vi "Parameters To Technique Parameters.vi"(8 "error in (no error)":errorcluster, 10 "Parameters":T1, 11 "ParameterIN":variant) -> (0 "error out":errorcluster, 3 "Params Values":T2[](array[typedef]))   [LabVIEW 2022 SP3, in "EClib functions.lvlib"]
uses:
  EClib functions.lvlib
  TechniqueParameters.ctl
  Parameters.ctl
  CAParameters.ctl
  CASGParameters.ctl
  CPParameters.ctl
  GEISParameters.ctl
  ISCANParameters.ctl
  OCVParameters.ctl
  PEISParameters.ctl
  SCCXParameters.ctl
  SGEISParameters.ctl
  SPEISParameters.ctl
  VSCANParameters.ctl
  MPParameters.ctl
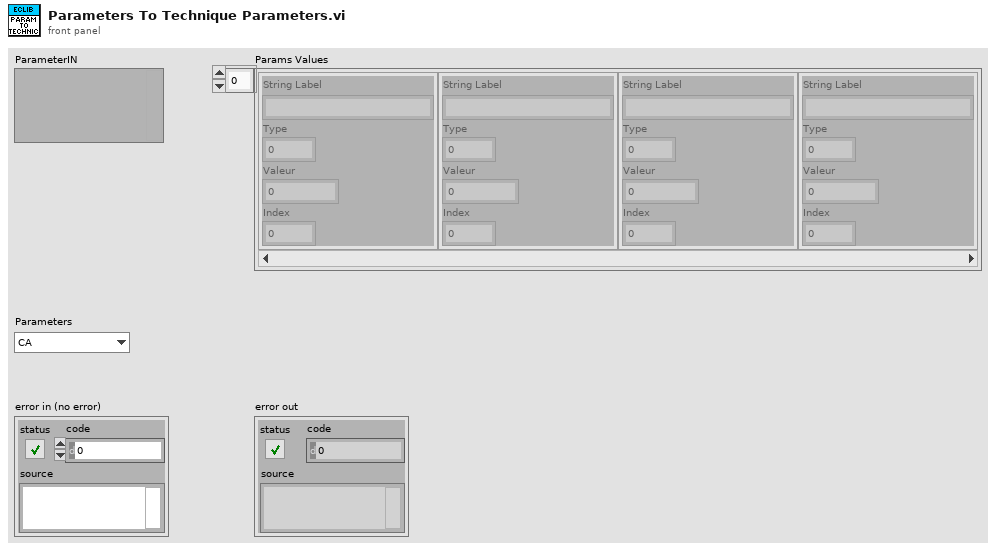
[diagram p1: front panel]
types:
  T1 = typedef "EClib functions.lvlib/Parameters.ctl" = enum16{"CA", "CASG", "CP", "GEIS", "ISCAN", "OCV", "PEIS", "SCCX", "SGEIS", "SPEIS", "VSCAN", "MP"}
  T2 = typedef "EClib functions.lvlib/TechniqueParameters.ctl" = cluster{"String Label":string, "Type":i32, "Valeur":i32, "Index":i32}
  T3 = typedef "EClib functions.lvlib/CAParameters.ctl" = cluster{"tb":sgl, "Steps":cluster{"vs_initial":bool, "Voltage_step":sgl, "Duration_step":sgl}[], "Step_number":i32, "N_Cycles":i32, "Record_every_dI":sgl, "Record_every_dT":sgl, "I_Range":u16, "E_Range":u16, "Bandwidth":u16, "em":u16, "ce":u16}
  T4 = typedef "EClib functions.lvlib/CASGParameters.ctl" = cluster{"Ii":sgl, "Ii_vs_initial":bool, "Steps":cluster{"I1_vs_initial":bool, "I1":sgl, "Period_number":u32, "Fs":sgl, "Record_every_dE":sgl, "Record_every_dT":sgl, "I2_vs_initial":bool, "I2":sgl}[], "Step_number":i32, "N_Cycles":i32, "I_Range":u16, "Bandwidth":u16, "em":u16, "ce":u16, "tb":sgl}
  T5 = typedef "EClib functions.lvlib/CPParameters.ctl" = cluster{"Steps":cluster{"vs_initial":bool, "Current_step":sgl, "Duration_step":sgl}[], "Step_number":i32, "N_Cycles":i32, "Record_every_dE":sgl, "Record_every_dT":sgl, "I_Range":u16, "E_Range":u16, "Bandwidth":u16, "em":u16, "ce":u16, "tb":sgl}
  T6 = typedef "EClib functions.lvlib/GEISParameters.ctl" = cluster{"Step_number":i32, "Initial_Current_step":sgl, "vs_initial ":bool, "Final_Current_step":sgl, "vs_final":bool, "Duration_step":sgl, "Record_every_dE":sgl, "Record_every_dT":sgl, "Initial_frequency":sgl, "sweep":bool, "Final_frequency":sgl, "Frequency_number":i32, "Amplitude_Current":sgl, "Wait_for_steady":sgl, "Average_N_times":i32, "Correction":bool, "I_Range":u16, "Bandwidth":u16, "em":u16, "ce":u16}
  T7 = typedef "EClib functions.lvlib/ISCANParameters.ctl" = cluster{"vs_initial ":bool, "Current_step":sgl, "Scans":cluster{" vs_initial":bool, "Current_step":sgl, "Scan_Rate":sgl}[], "Scan_number":i32, "N_Cycles":i32, "Record_every_dI":sgl, "Begin_measuring_E":sgl, "End_measuring_E":sgl, "I_Range":u16, "E_Range":u16, "Bandwidth":u16, "em":u16, "ce":u16, "tb":sgl}
  T8 = typedef "EClib functions.lvlib/OCVParameters.ctl" = cluster{"Rest_time_T":sgl, "Record_every_dE":sgl, "Record_every_dT":sgl, "E_Range":u16, "em":u16, "ce":u16, "tb":sgl}
  T9 = typedef "EClib functions.lvlib/PEISParameters.ctl" = cluster{"Step_number":i32, "Initial_Voltage_step":sgl, "vs_initial":bool, "Final_Voltage_step":sgl, "vs_final":bool, "Duration_step":sgl, "Record_every_dI":sgl, "Record_every_dT":sgl, "Initial_frequency":sgl, "sweep":bool, "Final_frequency":sgl, "Frequency_number":i32, "Amplitude_Voltage":sgl, "Wait_for_steady":sgl, "Average_N_times":i32, "Correction":bool, "I_Range":u16, "Bandwidth":u16, "em":u16, "ce":u16}
  T10 = typedef "EClib functions.lvlib/SCCXParameters.ctl" = cluster{"I_Range":u16, "E_Range":u16, "Bandwidth":u16, "par_E0":sgl, "par_A":sgl, "par_B":sgl, "par_QRP_select":u16, "par_E_duration":sgl, "par_E_dt_rec":sgl, "par_I0_duration":sgl, "par_I0_dt_rec":sgl, "par_NC":i32, "par_RC":i32, "par_Q_limit_val":sgl, "par_Q_limit_cfg":u16, "par_QRP_time":sgl, "ce":i32, "em":i32}
  T11 = cluster{"SCCX Parameters":T10, "Channel information":cluster{"Channel":i32, "BoardVersion":i32, "BoardSerialCode":i32, "FirmwareCode":i32, "FirmwareVersion":i32, "XilinxVersion":i32, "AmpCode":i32, "NbAmp":i32, "LcBoard":i32, "Zboard":i32, "MuxBoard":i32, "GPRAboard":i32, "MemSize":i32, "MemFilled":i32, "state":i32, "MaxIRange":i32, "MinIRange":i32, "MaxBandwidth":i32, "NbOfTechniques":i32}}
  T12 = typedef "EClib functions.lvlib/SGEISParameters.ctl" = cluster{"Step_number":i32, "Initial_Current_step":sgl, "vs_initial ":bool, "Final_Current_step":sgl, "vs_final":bool, "Duration_step":sgl, "Record_every_dE":sgl, "Record_every_dT":sgl, "Initial_frequency":sgl, "sweep":bool, "Final_frequency":sgl, "Frequency_number":i32, "Amplitude_Current":sgl, "Wait_for_steady":sgl, "Average_N_times":i32, "Correction":bool, "I_Range":u16, "Bandwidth":u16, "em":u16, "ce":u16}
  T13 = typedef "EClib functions.lvlib/SPEISParameters.ctl" = cluster{"Step_number":i32, "Initial_Voltage_step":sgl, "vs_initial":bool, "Final_Voltage_step":sgl, "vs_final":bool, "Duration_step":sgl, "Record_every_dI":sgl, "Record_every_dT":sgl, "Initial_frequency":sgl, "sweep":bool, "Final_frequency":sgl, "Frequency_number":i32, "Amplitude_Voltage":sgl, "Wait_for_steady":sgl, "Average_N_times":i32, "Correction":bool, "I_Range":u16, "Bandwidth":u16, "em":u16, "ce":u16}
  T14 = typedef "EClib functions.lvlib/VSCANParameters.ctl" = cluster{"tb":sgl, "vs_initial ":bool, "Voltage_step":sgl, "Scans":cluster{" vs_initial ":bool, "Voltage_step":sgl, "Scan_Rate":sgl}[], "Scan_number":i32, "N_Cycles":i32, "Record_every_dE":sgl, "Begin_measuring_I":sgl, "End_measuring_I":sgl, "I_Range":u16, "E_Range":u16, "Bandwidth":u16, "em":u16, "ce":u16}
  T15 = typedef "EClib functions.lvlib/MPParameters.ctl" = cluster{"tb":sgl, "Scans":cluster{"Value_step":sgl, "Duration_step":sgl, " vs_initial ":bool, "Record_every_dT":sgl, "Record_every_dM":sgl, "Mode_step":i32}[], "I_Range":u16, "Bandwidth":u16, "N_Cycles":i32, "Record_every_rc":i32, "ce":u16, "em":u16, "Step_number":i32}
  T16 = cluster{"I1_vs_initial":bool, "I1":sgl, "Period_number":u32, "Fs":sgl, "Record_every_dE":sgl, "Record_every_dT":sgl, "I2_vs_initial":bool, "I2":sgl}[]
  T17 = cluster{"I1_vs_initial":bool, "I1":sgl, "Period_number":u32, "Fs":sgl, "Record_every_dE":sgl, "Record_every_dT":sgl, "I2_vs_initial":bool, "I2":sgl}
  T18 = cluster{"Channel":i32, "BoardVersion":i32, "BoardSerialCode":i32, "FirmwareCode":i32, "FirmwareVersion":i32, "XilinxVersion":i32, "AmpCode":i32, "NbAmp":i32, "LcBoard":i32, "Zboard":i32, "MuxBoard":i32, "GPRAboard":i32, "MemSize":i32, "MemFilled":i32, "state":i32, "MaxIRange":i32, "MinIRange":i32, "MaxBandwidth":i32, "NbOfTechniques":i32}
  T19 = cluster{"Label":string, "type":i32, "valeur":u32, "index":i32}[]
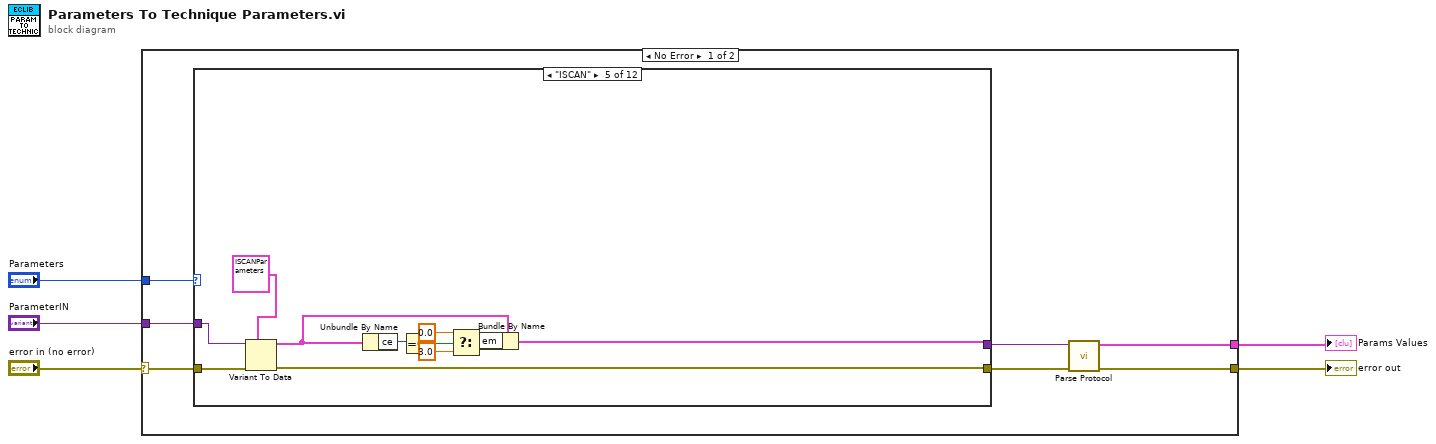
[diagram p0: block diagram]
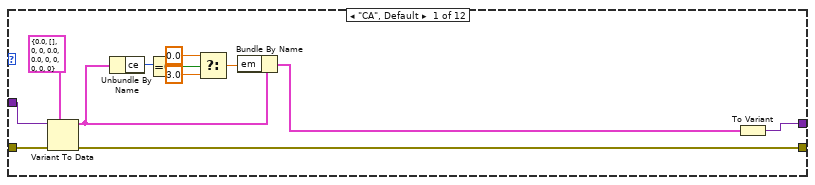
[diagram p2: hidden frame]
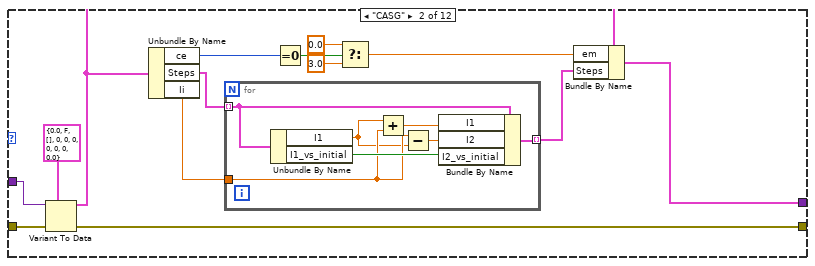
[diagram p3: hidden frame]
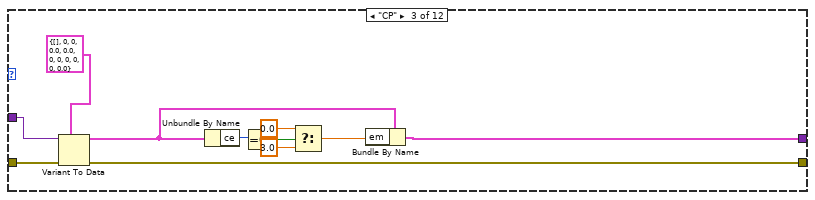
[diagram p4: hidden frame]
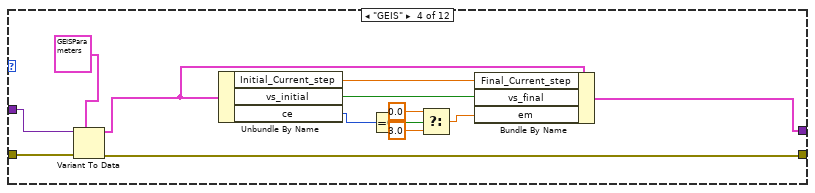
[diagram p5: hidden frame]
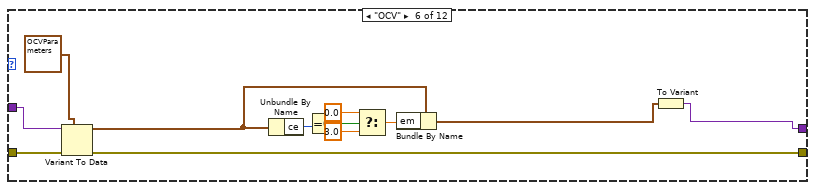
[diagram p6: hidden frame]
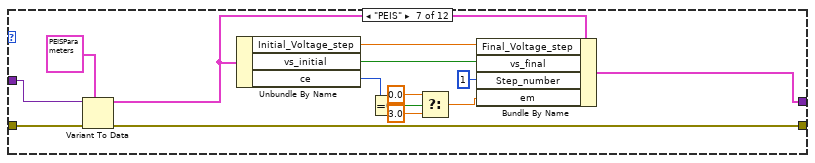
[diagram p7: hidden frame]
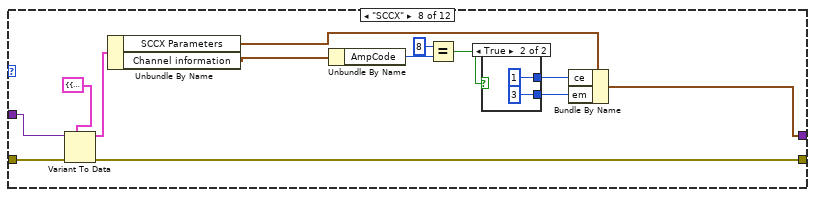
[diagram p8: hidden frame]
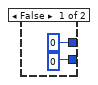
[diagram p9: hidden frame]
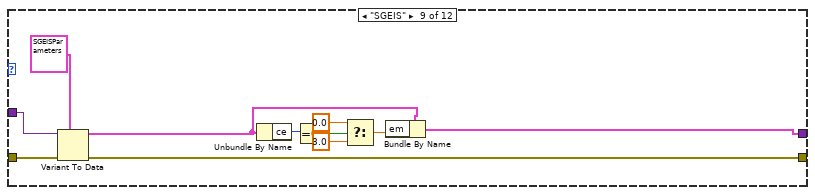
[diagram p10: hidden frame]
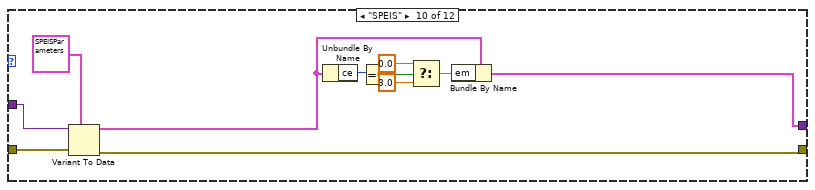
[diagram p11: hidden frame]
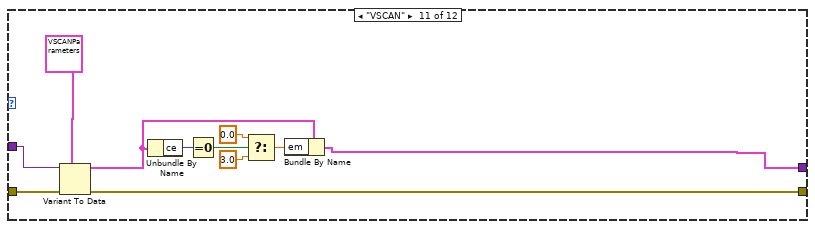
[diagram p12: hidden frame]
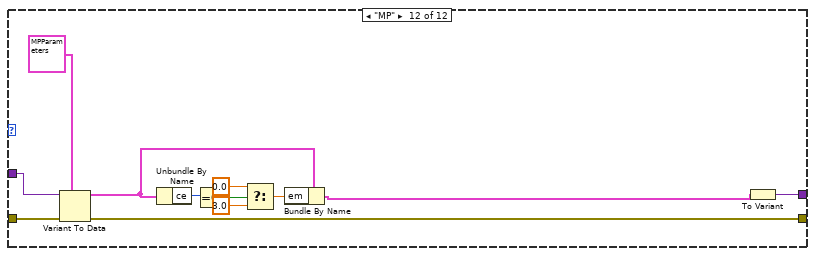
[diagram p13: hidden frame]
diagram:
  n1 = case shown="No Error" "error in (no error)" {
    selector: "error in (no error)" -> [w12 w169]
    tunnel: [w8 _] -> w5
    tunnel: [w6 w169] -> w3
    tunnel: "ParameterIN" -> [w10 _]
    tunnel: "Parameters" -> [w11 _]
    frame No Error {
      n2 = case shown="\"ISCAN\"" w11 {
        tunnel: [w14 w26 w47 w58 w70 w81 w94 w108 w124 w135 w146 w157] -> w9
        tunnel: w12 -> [w19 w38 w51 w69 w80 w92 w105 w119 w134 w145 w156 w168]
        tunnel: w10 -> [w17 w37 w50 w68 w79 w91 w106 w118 w133 w144 w155 w167]
        tunnel: [w13 w25 w46 w66 w77 w89 w93 w107 w132 w143 w147 w166] -> w7
        frame "CA", Default {
          n3 = Variant To Data(error in=w19, type=T3 {"tb"=0.0, "Steps"=[], "Step_number"=0, "N_Cycles"=0, "Record_every_dI"=0.0, "Record_every_dT"=0.0, "I_Range"=0, "E_Range"=0, "Bandwidth"=0, "em"=0, "ce"=0} ("CA Parameters"), Variant=w17) -> (data=w16:T3, error out=w13:errorcluster)
          n4 = Unbundle By Name(w16) -> ("ce"=w23:u16)
          n5 = Equal To 0?(x=w23) -> (x = 0?=w24:bool)
          n6 = Select(t=0.0, s=w24, f=3.0) -> (s? t:f=w20:dbl)
          n7 = Bundle By Name(cluster=w16, "em"=w20) -> (w15:T3)
          n8 = To Variant(anything=w15) -> (Variant=w14:variant)
        }
        frame "CASG" {
          n9 = Variant To Data(error in=w38, type=T4 {"Ii"=0.0, "Ii_vs_initial"=FALSE, "Steps"=[], "Step_number"=0, "N_Cycles"=0, "I_Range"=0, "Bandwidth"=0, "em"=0, "ce"=0, "tb"=0.0} ("CASG  Parameters"), Variant=w37) -> (data=w27:T4, error out=w25:errorcluster)
          n10 = Unbundle By Name(w27) -> ("ce"=w31:u16, "Steps"=w34:T16, "Ii"=w35:sgl)
          n11 = for {
            tunnel: [w45] -> w33 mode=indexing
            tunnel: w34 -> [w43] mode=indexing
            tunnel: w35 -> [w40]
            n12 = Unbundle By Name(w43) -> ("I1"=w39:sgl, "I1_vs_initial"=w44:bool)
            n13 = Add(x=w39, y=w40) -> (x+y=w42:sgl)
            n14 = Subtract(x=w40, y=w39) -> (x-y=w41:sgl)
            n15 = Bundle By Name(cluster=w43, "I1"=w42, "I2"=w41, "I2_vs_initial"=w44) -> (w45:T17)
          }
          n16 = Equal To 0?(x=w31) -> (x = 0?=w30:bool)
          n17 = Select(t=0.0, s=w30, f=3.0) -> (s? t:f=w32:dbl)
          n18 = Bundle By Name(cluster=w27, "em"=w32, "Steps"=w33) -> (w26:T4)
        }
        frame "CP" {
          n19 = Variant To Data(error in=w51, type=T5 {"Steps"=[], "Step_number"=0, "N_Cycles"=0, "Record_every_dE"=0.0, "Record_every_dT"=0.0, "I_Range"=0, "E_Range"=0, "Bandwidth"=0, "em"=0, "ce"=0, "tb"=0.0} ("CP Parameters"), Variant=w50) -> (data=w48:T5, error out=w46:errorcluster)
          n20 = Unbundle By Name(w48) -> ("ce"=w55:u16)
          n21 = Equal To 0?(x=w55) -> (x = 0?=w56:bool)
          n22 = Select(t=0.0, s=w56, f=3.0) -> (s? t:f=w52:dbl)
          n23 = Bundle By Name(cluster=w48, "em"=w52) -> (w47:T5)
        }
        frame "GEIS" {
          n24 = Variant To Data(error in=w69, type=T6 {"Step_number"=0, "Initial_Current_step"=0.0, "vs_initial "=FALSE, "Final_Current_step"=0.0, "vs_final"=FALSE, "Duration_step"=0.0, "Record_every_dE"=0.0, "Record_every_dT"=0.0, "Initial_frequency"=0.0, "sweep"=FALSE, "Final_frequency"=0.0, "Frequency_number"=0, "Amplitude_Current"=0.0, "Wait_for_steady"=0.0, "Average_N_times"=0, "Correction"=FALSE, "I_Range"=0, "Bandwidth"=0, "em"=0, "ce"=0} ("GEIS Parameters"), Variant=w68) -> (data=w57:T6, error out=w66:errorcluster)
          n25 = Unbundle By Name(w57) -> ("Initial_Current_step"=w59:sgl, "vs_initial"=w60:bool, "ce"=w64:u16)
          n26 = Equal To 0?(x=w64) -> (x = 0?=w63:bool)
          n27 = Select(t=0.0, s=w63, f=3.0) -> (s? t:f=w65:dbl)
          n28 = Bundle By Name(cluster=w57, "Final_Current_step"=w59, "vs_final"=w60, "em"=w65) -> (w58:T6)
        }
        frame "ISCAN" {
          n29 = Variant To Data(error in=w80, type=T7 {"vs_initial "=FALSE, "Current_step"=0.0, "Scans"=[], "Scan_number"=0, "N_Cycles"=0, "Record_every_dI"=0.0, "Begin_measuring_E"=0.0, "End_measuring_E"=0.0, "I_Range"=0, "E_Range"=0, "Bandwidth"=0, "em"=0, "ce"=0, "tb"=0.0} ("ISCAN Parameters"), Variant=w79) -> (data=w71:T7, error out=w77:errorcluster)
          n30 = Unbundle By Name(w71) -> ("ce"=w75:u16)
          n31 = Equal To 0?(x=w75) -> (x = 0?=w76:bool)
          n32 = Select(t=0.0, s=w76, f=3.0) -> (s? t:f=w72:dbl)
          n33 = Bundle By Name(cluster=w71, "em"=w72) -> (w70:T7)
        }
        frame "OCV" {
          n34 = Variant To Data(error in=w92, type=T8 {"Rest_time_T"=1.0, "Record_every_dE"=0.01, "Record_every_dT"=0.01, "E_Range"=3, "em"=1, "ce"=0, "tb"=2e-05} ("OCV Parameters"), Variant=w91) -> (data=w83:T8, error out=w89:errorcluster)
          n35 = Unbundle By Name(w83) -> ("ce"=w87:u16)
          n36 = Equal To 0?(x=w87) -> (x = 0?=w88:bool)
          n37 = Select(t=0.0, s=w88, f=3.0) -> (s? t:f=w84:dbl)
          n38 = Bundle By Name(cluster=w83, "em"=w84) -> (w82:T8)
          n39 = To Variant(anything=w82) -> (Variant=w81:variant)
        }
        frame "PEIS" {
          n40 = Variant To Data(error in=w105, type=T9 {"Step_number"=0, "Initial_Voltage_step"=0.0, "vs_initial"=FALSE, "Final_Voltage_step"=0.0, "vs_final"=FALSE, "Duration_step"=0.0, "Record_every_dI"=0.0, "Record_every_dT"=0.0, "Initial_frequency"=0.0, "sweep"=FALSE, "Final_frequency"=0.0, "Frequency_number"=0, "Amplitude_Voltage"=0.0, "Wait_for_steady"=0.0, "Average_N_times"=0, "Correction"=FALSE, "I_Range"=0, "Bandwidth"=0, "em"=0, "ce"=0} ("PEIS Parameters"), Variant=w106) -> (data=w95:T9, error out=w93:errorcluster)
          n41 = Unbundle By Name(w95) -> ("Initial_Voltage_step"=w96:sgl, "vs_initial"=w97:bool, "ce"=w102:u16)
          n42 = Equal To 0?(x=w102) -> (x = 0?=w101:bool)
          n43 = Select(t=0.0, s=w101, f=3.0) -> (s? t:f=w103:dbl)
          n44 = Bundle By Name(cluster=w95, "Final_Voltage_step"=w96, "vs_final"=w97, "Step_number"=1, "em"=w103) -> (w94:T9)
        }
        frame "SCCX" {
          n45 = Variant To Data(error in=w119, type=T11 {"SCCX Parameters"={"I_Range"=11, "E_Range"=0, "Bandwidth"=3, "par_E0"=1.0, "par_A"=0.0, "par_B"=0.1, "par_QRP_select"=1, "par_E_duration"=0.01, "par_E_dt_rec"=0.0001, "par_I0_duration"=0.01, "par_I0_dt_rec"=0.0001, "par_NC"=9, "par_RC"=1, "par_Q_limit_val"=5e-05, "par_Q_limit_cfg"=0, "par_QRP_time"=0.005, "ce"=0, "em"=0}, "Channel information"={"Channel"=0, "BoardVersion"=0, "BoardSerialCode"=0, "FirmwareCode"=0, "FirmwareVersion"=0, "XilinxVersion"=0, "AmpCode"=0, "NbAmp"=0, "LcBoard"=0, "Zboard"=0, "MuxBoard"=0, "GPRAboard"=0, "MemSize"=0, "MemFilled"=0, "state"=0, "MaxIRange"=0, "MinIRange"=0, "MaxBandwidth"=0, "NbOfTechniques"=0}}, Variant=w118) -> (data=w116:T11, error out=w107:errorcluster)
          n46 = Unbundle By Name(w116) -> ("SCCX Parameters"=w109:T10, "Channel information"=w110:T18)
          n47 = Unbundle By Name(w110) -> ("AmpCode"=w112:i32)
          n48 = Equal?(x=8, y=w112) -> (x = y?=w111:bool)
          n49 = case shown="True" w111 {
            tunnel: [0 ("ce") 1 ("ce")] -> w114
            tunnel: [0 ("ce") 3 ("ce")] -> w115
            frame False {
            }
            frame True {
            }
          }
          n50 = Bundle By Name(cluster=w109, "ce"=w114, "em"=w115) -> (w108:T10)
        }
        frame "SGEIS" {
          n51 = Variant To Data(error in=w134, type=T12 {"Step_number"=0, "Initial_Current_step"=0.0, "vs_initial "=FALSE, "Final_Current_step"=0.0, "vs_final"=FALSE, "Duration_step"=0.0, "Record_every_dE"=0.0, "Record_every_dT"=0.0, "Initial_frequency"=0.0, "sweep"=FALSE, "Final_frequency"=0.0, "Frequency_number"=0, "Amplitude_Current"=0.0, "Wait_for_steady"=0.0, "Average_N_times"=0, "Correction"=FALSE, "I_Range"=0, "Bandwidth"=0, "em"=0, "ce"=0} ("SGEIS Parameters"), Variant=w133) -> (data=w125:T12, error out=w132:errorcluster)
          n52 = Unbundle By Name(w125) -> ("ce"=w129:u16)
          n53 = Equal To 0?(x=w129) -> (x = 0?=w130:bool)
          n54 = Select(t=0.0, s=w130, f=3.0) -> (s? t:f=w126:dbl)
          n55 = Bundle By Name(cluster=w125, "em"=w126) -> (w124:T12)
        }
        frame "SPEIS" {
          n56 = Variant To Data(error in=w145, type=T13 {"Step_number"=0, "Initial_Voltage_step"=0.0, "vs_initial"=FALSE, "Final_Voltage_step"=0.0, "vs_final"=FALSE, "Duration_step"=0.0, "Record_every_dI"=0.0, "Record_every_dT"=0.0, "Initial_frequency"=0.0, "sweep"=FALSE, "Final_frequency"=0.0, "Frequency_number"=0, "Amplitude_Voltage"=0.0, "Wait_for_steady"=0.0, "Average_N_times"=0, "Correction"=FALSE, "I_Range"=0, "Bandwidth"=0, "em"=0, "ce"=0} ("SPEIS Parameters"), Variant=w144) -> (data=w136:T13, error out=w143:errorcluster)
          n57 = Unbundle By Name(w136) -> ("ce"=w140:u16)
          n58 = Equal To 0?(x=w140) -> (x = 0?=w141:bool)
          n59 = Select(t=0.0, s=w141, f=3.0) -> (s? t:f=w137:dbl)
          n60 = Bundle By Name(cluster=w136, "em"=w137) -> (w135:T13)
        }
        frame "VSCAN" {
          n61 = Variant To Data(error in=w156, type=T14 {"tb"=0.0, "vs_initial "=FALSE, "Voltage_step"=0.0, "Scans"=[], "Scan_number"=0, "N_Cycles"=0, "Record_every_dE"=0.0, "Begin_measuring_I"=0.0, "End_measuring_I"=0.0, "I_Range"=0, "E_Range"=0, "Bandwidth"=0, "em"=0, "ce"=0} ("VSCAN Parameters"), Variant=w155) -> (data=w148:T14, error out=w147:errorcluster)
          n62 = Unbundle By Name(w148) -> ("ce"=w151:u16)
          n63 = Equal To 0?(x=w151) -> (x = 0?=w152:bool)
          n64 = Select(t=0.0, s=w152, f=3.0) -> (s? t:f=w149:dbl)
          n65 = Bundle By Name(cluster=w148, "em"=w149) -> (w146:T14)
        }
        frame "MP" {
          n66 = Variant To Data(error in=w168, type=T15 {"tb"=5e-05, "Scans"=[], "I_Range"=12, "Bandwidth"=5, "N_Cycles"=0, "Record_every_rc"=0, "ce"=0, "em"=1, "Step_number"=0} ("MP Parameters"), Variant=w167) -> (data=w160:T15, error out=w166:errorcluster)
          n67 = Unbundle By Name(w160) -> ("ce"=w163:u16)
          n68 = Equal To 0?(x=w163) -> (x = 0?=w164:bool)
          n69 = Select(t=0.0, s=w164, f=3.0) -> (s? t:f=w159:dbl)
          n70 = Bundle By Name(cluster=w160, "em"=w159) -> (w158:T15)
          n71 = To Variant(anything=w158) -> (Variant=w157:variant)
        }
      }
      n72 = call "Parse Protocol.vi"("error in (no error)"=w7, "Protocol Cluster"=w9) -> ("error out"=w6:errorcluster, "Params Values"=w8:T19)  [unwired: 8 in]
    }
    frame Error {
    }
  }
  "Params Values" <- w5
  "error out" <- w3
